vi "rep_cap_add.vi"(7 "Rep Cap Name":string, 8 "error in":errorcluster, 9 "Command Value":string, 10 "Rep Cap Name ID":string, 11 "VISA resource name":refnum<visa-resource-name>) -> (0 "error out":errorcluster, 3 "VISA resource name out":refnum<visa-resource-name>)   [LabVIEW 2014, in "rszvl_rsidr_core.lvlib"]
uses:
  rszvl_rsidr_core.lvlib
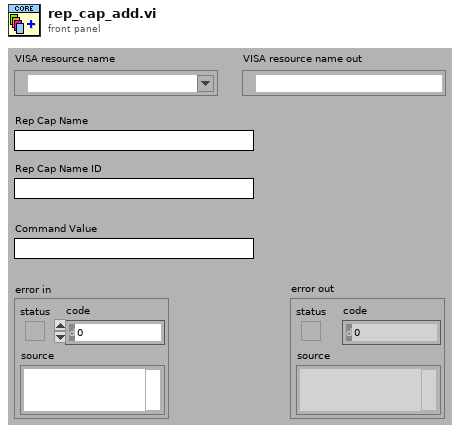
[diagram p1: front panel]
types:
  T1 = enum16{"Initialize", "Get Cmd Value", "Reset Rep Cap", "Add Rep Cap", "Remove Rep Cap", "Get Rep Cap ID range", "Get Count", "Clear", "Find Name from NameID", "Get First NameID"}
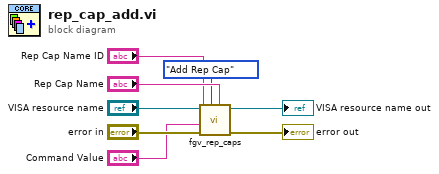
[diagram p0: block diagram]
diagram:
  n1 = call "fgv_rep_caps.vi"("RepCapName in (\"\")"="Rep Cap Name", "Operation"=T1."Add Rep Cap", "error in"="error in", "RepCapNameCmdValue in (\"\")"="Command Value", "RepCapNameID in (\"\")"="Rep Cap Name ID", "VISA resource name"="VISA resource name") -> ("error out"=→"error out":errorcluster, "VISA resource name out"=→"VISA resource name out":refnum<visa-resource-name>)  [unwired: 2 in, 2 out]
